vi "myRIO_BRig_Host_comm_webdav_uploadSettings.vi"(11 "input_filePath":path) -> ()   [LabVIEW 2014]
uses:
  <vilib>/WebDAVClient/NI_WebDAV.lvlib
panel:
  out "error out 3":errorcluster
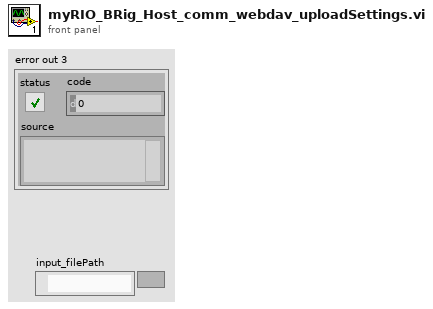
[diagram p1: front panel]
types:
  T1 = typedef "NI_WebDAV.lvlib/SessionHandle.ctl" = refnum<k1>
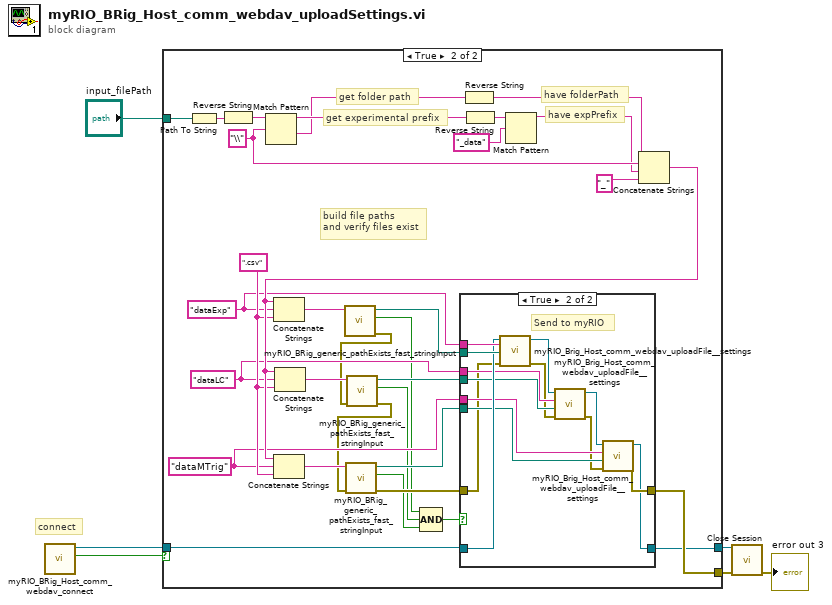
[diagram p0: block diagram]
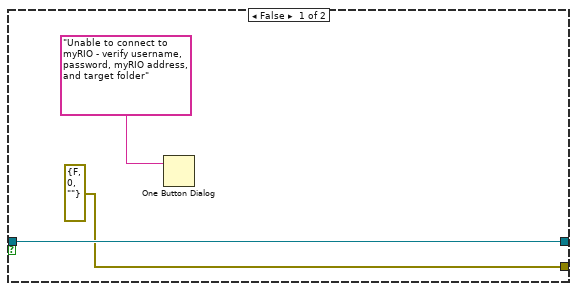
[diagram p2: hidden frame]
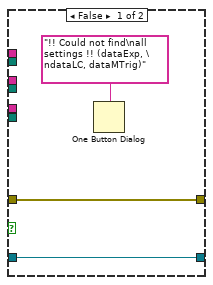
[diagram p3: hidden frame]
diagram:
  # "connect"
  n1 = call "myRIO_BRig_Host_comm_webdav_connect.vi"() -> ("output_Iconnected"=w4:bool, "output_hSession"=w5:T1)  [unwired: 9 in, 1 out]
  n2 = case shown="True" w4 {
    tunnel: "input_filePath" -> [_ w41]
    tunnel: w5 -> [w8 w28]
    tunnel: [w8 w13] -> w2
    tunnel: [errorcluster {"status"=FALSE, "code"=0, "source"=""} ("error in (no error)") w14] -> w1
    frame False {
      n3 = One Button Dialog(message="Unable to connect to myRIO - verify username, password, myRIO address, and target folder" ("t")) -> ()  [unwired: 1 in, 1 out]
    }
    frame True {
      w25 = "dataMTrig" ("regular expression")
      w26 = "dataLC" ("regular expression")
      w29 = ".csv" ("string")
      w27 = "dataExp" ("regular expression")
      w33 = "\\" ("regular expression")
      # "build file paths\nand verify files exist"
      # "get folder path"
      # "get experimental prefix"
      # "have expPrefix"
      # "have folderPath"
      n4 = Path To String(path=w41) -> (string=w40:string)
      n5 = Reverse String(1:w40) -> (0:w39:string)
      n6 = Match Pattern(string=w39, regular expression=w33) -> (before substring=w38:string, after substring=w35:string)  [unwired: 1 in, 2 out]
      n7 = Reverse String(1:w35) -> (0:w34:string)
      n8 = Reverse String(1:w38) -> (0:w37:string)
      n9 = Match Pattern(string=w37, regular expression="_data") -> (before substring=w32:string)  [unwired: 1 in, 3 out]
      n10 = Concatenate Strings(w34, w33, w32, "_" ("string")) -> (w30:string)
      n11 = Concatenate Strings(w30, w27, w29) -> (w23:string)
      n12 = Concatenate Strings(w30, w25, w29) -> (w19:string)
      n13 = Concatenate Strings(w30, w26, w29) -> (w21:string)
      n14 = call "myRIO_BRig_generic_pathExists_fast_stringInput.vi"("input_filePath"=w23) -> ("output_error"=w17:errorcluster, "output_Iexist"=w10:bool, "output_filePath"=w22:path)  [unwired: 8 in]
      n15 = call "myRIO_BRig_generic_pathExists_fast_stringInput.vi"("input_error"=w17, "input_filePath"=w21) -> ("output_error"=w16:errorcluster, "output_Iexist"=w11:bool, "output_filePath"=w20:path)  [unwired: 7 in]
      n16 = call "myRIO_BRig_generic_pathExists_fast_stringInput.vi"("input_error"=w16, "input_filePath"=w19) -> ("output_error"=w15:errorcluster, "output_Iexist"=w12:bool, "output_filePath"=w18:path)  [unwired: 7 in]
      n17 = Compound Arithmetic op=AND(w10, w11, w12) -> (w24:bool)
      n18 = case shown="True" w24 {
        tunnel: w22 -> [_ w58]
        tunnel: w20 -> [_ w53]
        tunnel: w18 -> [_ w50]
        tunnel: w28 -> [w43 w56]
        tunnel: w27 -> [_ w57]
        tunnel: w26 -> [_ w54]
        tunnel: w25 -> [_ w51]
        tunnel: w15 -> [w42 w47]
        tunnel: [w43 w45] -> w13
        tunnel: [w42 w46] -> w14
        frame False {
          n19 = One Button Dialog(message="!! Could not find\nall settings !! (dataExp, \ndataLC, dataMTrig)") -> ()  [unwired: 1 in, 1 out]
        }
        frame True {
          # "Send to myRIO"
          n20 = call "myRIO_Brig_Host_comm_webdav_uploadFile__settings.vi"("input_error"=w47, "input_filePath_local"=w58, "dataName"=w57, "input_hSession"=w56) -> ("output_error"=w49:errorcluster, "output_hSession"=w55:T1)  [unwired: 5 in, 1 out]
          n21 = call "myRIO_Brig_Host_comm_webdav_uploadFile__settings.vi"("input_error"=w49, "input_filePath_local"=w53, "dataName"=w54, "input_hSession"=w55) -> ("output_error"=w48:errorcluster, "output_hSession"=w52:T1)  [unwired: 5 in, 1 out]
          n22 = call "myRIO_Brig_Host_comm_webdav_uploadFile__settings.vi"("input_error"=w48, "input_filePath_local"=w50, "dataName"=w51, "input_hSession"=w52) -> ("output_error"=w46:errorcluster, "output_hSession"=w45:T1)  [unwired: 5 in, 1 out]
        }
      }
    }
  }
  n23 = call <vilib>:"Close Session.vi"("session handle"=w2, "error in (no error)"=w1) -> ("error out"=→"error out 3":errorcluster)  [unwired: 13 in]
